vi "CalibrationsGlobalVariables.vi"() -> ()   [LabVIEW 2019]
uses:
  <vilib>/Rock Robotics/WPI/Solenoid/WPI_SolenoidValue.ctl
panel:
  out "ReadToWrite":bool=TRUE
  in  "time_to_run":u32
  in  "Spinwheel_Throttle":dbl
  in  "Top_IR_Threshold":dbl
  in  "Bottom_Middle_IR_Threshold":dbl=1.5
  in  "Top_Middle_IR_Threshold":dbl=2.0
  in  "Bottom_IR_Threshold":dbl
  in  "Intake_Speed":dbl
  in  "Firing_Speed":dbl=1.0
  in  "Max Magazine Speed":dbl=1050.0
  in  "Unjam_Speed":dbl
  in  "Loading_Speed":dbl=1.0
  in  "Intake Input":T1=enum."Reverse"
  in  "Hopper Input":T1=enum."Reverse"
  in  "extend delay(ms)":dbl=1000.0
  in  "retract delay(ms)":dbl=1000.0
  # "intake"
  # "magazine"
  # "control panel"
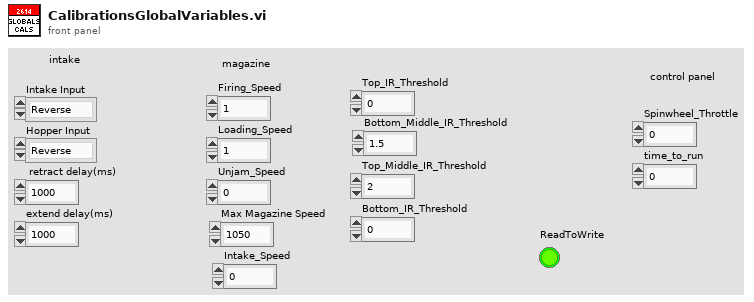
[diagram p1: front panel]
types:
  T1 = typedef "WPI_SolenoidValue.ctl" = enum16{"Off", "On", "Forward", "Reverse"}
diagram:
